vi "Set Write Timeout.vi"(8 "error in (no error)":errorcluster, 10 "write operation timeout":i32=5000, 11 "Modbus master in":refnum<class "Network Master.lvclass">) -> (0 "error out":errorcluster, 3 "Modbus master out":refnum<class "Network Master.lvclass">)   [LabVIEW 2021, in "Network Master.lvclass"]
doc: "<B>Write Timeout</B> specifies the write operation timeout. You can use a Modbus master instance to perform write operations on a Modbus slave with the specified timeout."
uses:
  Network Master.lvclass
  C:/my_projects/projects/Algorithms/Labview/21/Modbus_v121c/Network Protocol/Network Protocol.lvclass
  Network Protocol.lvclass/Network Protocol.ctl
  Transmission Data Unit/Transmission Data Unit.lvclass/Transmission Data Unit.ctl
  Network Master.lvclass/Network Master.ctl
  Transmission Data Unit/Transmission Data Unit.lvclass
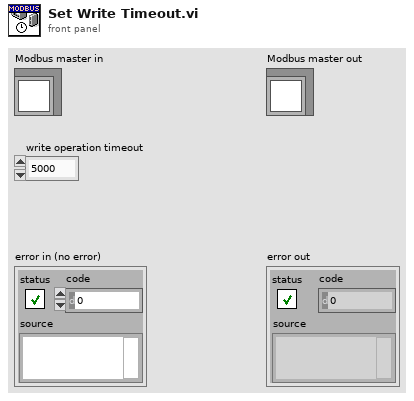
[diagram p1: front panel]
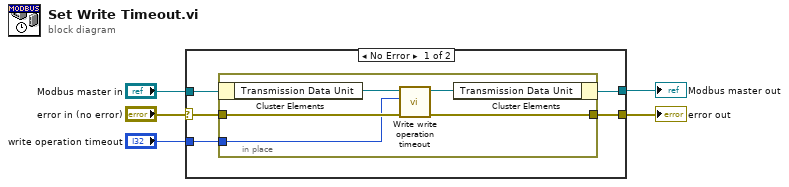
[diagram p0: block diagram]
diagram:
  n1 = case shown="No Error" "error in (no error)" {
    selector: "error in (no error)" -> [w8 w16]
    tunnel: "write operation timeout" -> [w6 _]
    tunnel: [w9 w17] -> w2
    tunnel: "Modbus master in" -> [w10 w17]
    tunnel: [w7 w16] -> w1
    frame No Error {
      n2 = in-place {
        in-place-border: w8 -> [w14]
        in-place-border: [w15] -> w7
        in-place-border: w6 -> [w11]
        n3 = in-place-cluster #1(w10) -> ("Transmission Data Unit"=w12:refnum<class "Transmission Data Unit.lvclass">)
        n4 = call "Write write operation timeout.vi"("error in (no error)"=w14, "write operation timeout"=w11, "transmission data unit in"=w12) -> ("error out"=w15:errorcluster, "transmission data unit out"=w13:refnum<class "Transmission Data Unit.lvclass">)  [unwired: 7 in]
        n5 = in-place-cluster #1("Transmission Data Unit"=w13) -> (w9:refnum<class "Network Master.lvclass">)
      }
    }
    frame Error {
    }
  }
  "error out" <- w1
  "Modbus master out" <- w2
